vi "globalTearDown.vi"(8 "error in (no error)":errorcluster, 11 "testcase-CSMStatus in":refnum<class "testcase-CSMBroadcast.lvclass">) -> (0 "error out":errorcluster, 3 "testcase-CSMStatus out":refnum<class "testcase-CSMBroadcast.lvclass">)   [LabVIEW 2017, in "testcase-CSMBroadcast.lvclass"]
uses:
  testcase-CSMBroadcast.lvclass
  testcase-CSMBroadcast.lvclass/testcase-CSMBroadcast.ctl
  <vilib>/addons/_JKI Toolkits/VI Tester/TestCase.llb/TestCase.lvclass
  src/user.lib/_NEVSTOP/Communicable State Machine(CSM)/_Support/Typedef/_CSM_List Module Scope.ctl
  src/user.lib/_NEVSTOP/Communicable State Machine(CSM)/Communicable State Machine.lvlib
panel:
  out "Module Names":string[](array[string])
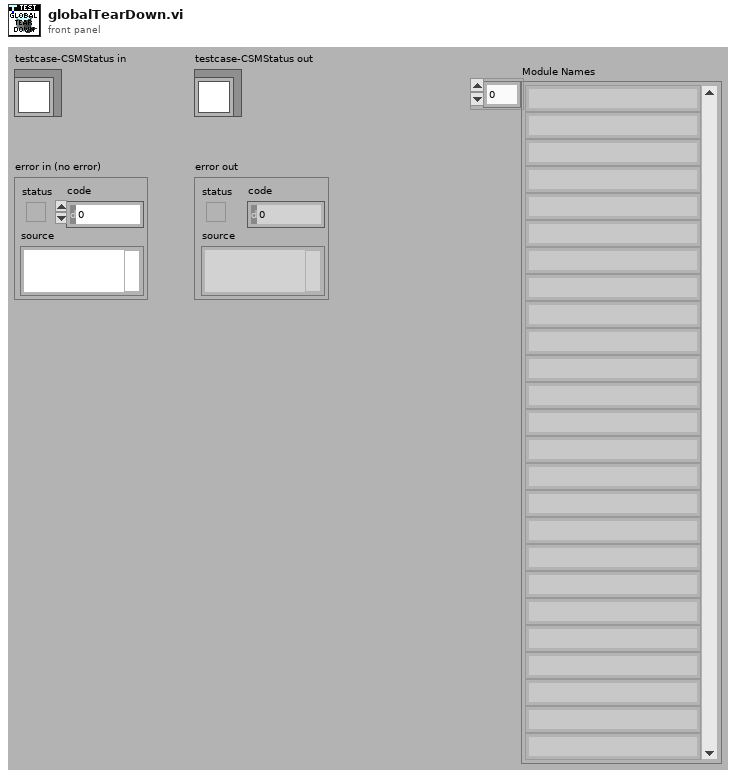
[diagram p1: front panel]
types:
  T1 = typedef "Communicable State Machine.lvlib/_CSM_List Module Scope.ctl" = enum16{"Normal", "System Only", "All"}
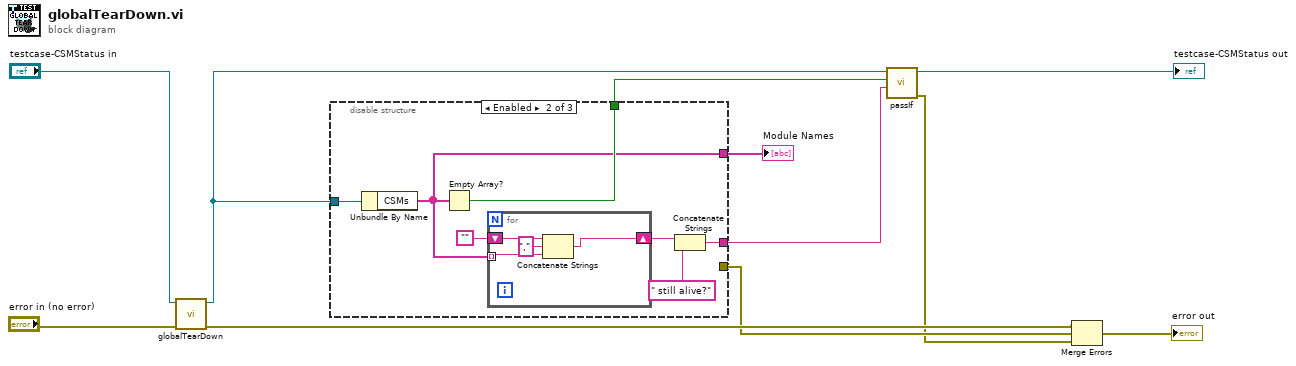
[diagram p0: block diagram]
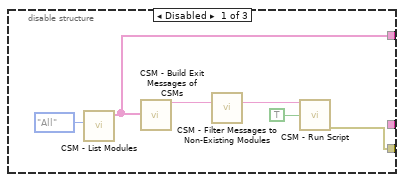
[diagram p2: hidden frame]
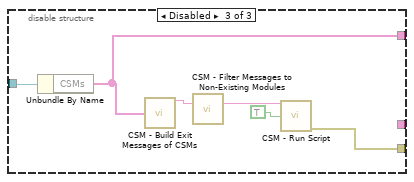
[diagram p3: hidden frame]
diagram:
  n1 = call-parent "globalTearDown.vi"("error in (no error)"="error in (no error)", "TestCase in"="testcase-CSMStatus in") -> ("error out"=w5:errorcluster, "TestCase out"=w1:refnum<class "testcase-CSMBroadcast.lvclass">)  [unwired: 8 in]
  n2 = disable-structure shown="Enabled" {
    disable-tunnel: [w13 _ w29] -> w4
    disable-tunnel: w1 -> [_ w24 w34]
    disable-tunnel: [w12 w22 w30] -> w8
    disable-tunnel: [_ w23 _] -> w7
    disable-tunnel: [_ w18 _] -> w6
    frame Disabled {
      n3 = call "CSM - List Modules.vi"("Scope (Normal)"=_CSM_List_Module_Scope."All") -> ("Module Names"=w12:string[])  [unwired: 9 in, 1 out]
      n4 = call "CSM - Build Exit Messages of CSMs.vi"("CSMs"=w12) -> ("States"=w17:string)  [unwired: 14 in]
      n5 = call "CSM - Filter Messages to Non-Existing Modules.vi"("States In"=w17) -> ("States Out"=w15:string)  [unwired: 14 in]
      n6 = call "CSM - Run Script.vi"("CSM Scripts"=w15, "Continue If Error? (F)"=TRUE) -> ("error out"=w13:errorcluster)  [unwired: 11 in, 2 out]
    }
    frame Enabled {
      n7 = Unbundle By Name(w24) -> ("CSMs"=w22:string[])
      n8 = Empty Array?(array=w22) -> (empty?=w23:bool)
      n9 = for {
        tunnel: w22 -> [w26] mode=indexing
        shift-right: [w27] -> w20
        shift-left: "" -> [w28]
        n10 = Concatenate Strings(w28, "," ("string"), w26) -> (w27:string)
      }
      n11 = Concatenate Strings(w20, " still alive?" ("string")) -> (w18:string)
    }
    frame Disabled {
      n12 = Unbundle By Name(w34) -> ("CSMs"=w30:string[])
      n13 = call "CSM - Build Exit Messages of CSMs.vi"("CSMs"=w30) -> ("States"=w33:string)  [unwired: 14 in]
      n14 = call "CSM - Filter Messages to Non-Existing Modules.vi"("States In"=w33) -> ("States Out"=w31:string)  [unwired: 14 in]
      n15 = call "CSM - Run Script.vi"("CSM Scripts"=w31, "Continue If Error? (F)"=TRUE) -> ("error out"=w29:errorcluster)  [unwired: 11 in, 2 out]
    }
  }
  "Module Names" <- w8
  n16 = call-dynamic "passIf.vi"("message (\"\")"=w6, "pass"=w7, "TestCase in"=w1) -> ("error out"=w3:errorcluster, "TestCase out"=→"testcase-CSMStatus out":refnum<class "testcase-CSMBroadcast.lvclass">)  [unwired: 7 in]
  n17 = Merge Errors(w5, w4, w3) -> (→"error out":errorcluster)
